vi "ProfilerTest.vi"() -> ()   [LabVIEW 2014] (continued)
{35.59000000000149, 1.3677623388053117e-07}, {35.60000000000149, 1.3677623388053117e-07}, {35.610000000001484, 1.3677623388053117e-07}, {35.62000000000148, 1.3677623388053117e-07}, {35.63000000000148, 1.3677623388053117e-07}, {35.64000000000148, 1.3677623388053117e-07}, {35.65000000000148, 1.3677623388053117e-07}, {35.660000000001475, 1.3677623388053117e-07}, {35.67000000000147, 1.3677623388053117e-07}, {35.68000000000147, 1.3677623388053117e-07}, {35.69000000000147, 1.3677623388053117e-07}, {35.70000000000147, 1.3677623388053117e-07}, {35.710000000001465, 1.3677623388053117e-07}, {35.72000000000146, 1.3677623388053117e-07}, {35.73000000000146, 1.3677623388053117e-07}, {35.74000000000146, 1.3677623388053117e-07}, {35.75000000000146, 1.3677623388053117e-07}, {35.760000000001455, 1.3677623388053117e-07}, {35.77000000000145, 1.3677623388053117e-07}, {35.78000000000145, 1.3677623388053117e-07}, {35.79000000000145, 1.3677623388053117e-07}, {35.80000000000145, 1.3677623388053117e-07}, {35.810000000001445, 1.3677623388053117e-07}, {35.82000000000144, 1.3677623388053117e-07}, {35.83000000000144, 1.3677623388053117e-07}, {35.84000000000144, 1.3677623388053117e-07}, {35.85000000000144, 1.3677623388053117e-07}, {35.860000000001435, 1.3677623388053117e-07}, {35.87000000000143, 1.3677623388053117e-07}, {35.88000000000143, 1.3677623388053117e-07}, {35.89000000000143, 1.3677623388053117e-07}, {35.90000000000143, 1.3677623388053117e-07}, {35.910000000001425, 1.3677623388053117e-07}, {35.92000000000142, 1.3677623388053117e-07}, {35.93000000000142, 1.3677623388053117e-07}, {35.94000000000142, 1.3677623388053117e-07}, {35.95000000000142, 1.3677623388053117e-07}, {35.960000000001415, 1.3677623388053117e-07}, {35.97000000000141, 1.3677623388053117e-07}, {35.98000000000141, 1.3677623388053117e-07}, {35.99000000000141, 1.3677623388053117e-07}, {36.00000000000141, 1.3677623388053117e-07}, {36.010000000001405, 1.3677623388053117e-07}, {36.0200000000014, 1.3677623388053117e-07}, {36.0300000000014, 1.3677623388053117e-07}, {36.0400000000014, 1.3677623388053117e-07}, {36.0500000000014, 1.3677623388053117e-07}, {36.060000000001395, 1.3677623388053117e-07}, {36.07000000000139, 1.3677623388053117e-07}, {36.08000000000139, 1.3677623388053117e-07}, {36.09000000000139, 1.3677623388053117e-07}, {36.10000000000139, 1.3677623388053117e-07}, {36.110000000001385, 1.3677623388053117e-07}, {36.12000000000138, 1.3677623388053117e-07}, {36.13000000000138, 1.3677623388053117e-07}, {36.14000000000138, 1.3677623388053117e-07}, {36.15000000000138, 1.3677623388053117e-07}, {36.160000000001375, 1.3677623388053117e-07}, {36.17000000000137, 1.3677623388053117e-07}, {36.18000000000137, 1.3677623388053117e-07}, {36.19000000000137, 1.3677623388053117e-07}, {36.20000000000137, 1.3677623388053117e-07}, {36.210000000001365, 1.3677623388053117e-07}, {36.22000000000136, 1.3677623388053117e-07}, {36.23000000000136, 1.3677623388053117e-07}, {36.24000000000136, 1.3677623388053117e-07}, {36.25000000000136, 1.3677623388053117e-07}, {36.260000000001355, 1.3677623388053117e-07}, {36.27000000000135, 1.3677623388053117e-07}, {36.28000000000135, 1.3677623388053117e-07}, {36.29000000000135, 1.3677623388053117e-07}, {36.30000000000135, 1.3677623388053117e-07}, {36.310000000001345, 1.3677623388053117e-07}, {36.32000000000134, 1.3677623388053117e-07}, {36.33000000000134, 1.3677623388053117e-07}, {36.34000000000134, 1.3677623388053117e-07}, {36.35000000000134, 1.3677623388053117e-07}, {36.360000000001335, 1.3677623388053117e-07}, {36.37000000000133, 1.3677623388053117e-07}, {36.38000000000133, 1.3677623388053117e-07}, {36.39000000000133, 1.3677623388053117e-07}, {36.40000000000133, 1.3677623388053117e-07}, {36.410000000001325, 1.3677623388053117e-07}, {36.42000000000132, 1.3677623388053117e-07}, {36.43000000000132, 1.3677623388053117e-07}, {36.44000000000132, 1.3677623388053117e-07}, {36.45000000000132, 1.3677623388053117e-07}, {36.460000000001315, 1.3677623388053117e-07}, {36.47000000000131, 1.3677623388053117e-07}, {36.48000000000131, 1.3677623388053117e-07}, {36.49000000000131, 1.3677623388053117e-07}, {36.50000000000131, 1.3677623388053117e-07}, {36.510000000001305, 1.3677623388053117e-07}, {36.5200000000013, 1.3677623388053117e-07}, {36.5300000000013, 1.3677623388053117e-07}, {36.5400000000013, 1.3677623388053117e-07}, {36.5500000000013, 1.3677623388053117e-07}, {36.560000000001295, 1.3677623388053117e-07}, {36.57000000000129, 1.3677623388053117e-07}, {36.58000000000129, 1.3677623388053117e-07}, {36.59000000000129, 1.3677623388053117e-07}, {36.60000000000129, 1.3677623388053117e-07}, {36.610000000001286, 1.3677623388053117e-07}, {36.62000000000128, 1.3677623388053117e-07}, {36.63000000000128, 1.3677623388053117e-07}, {36.64000000000128, 1.3677623388053117e-07}, {36.65000000000128, 1.3677623388053117e-07}, {36.660000000001276, 1.3677623388053117e-07}, {36.670000000001274, 1.3677623388053117e-07}, {36.68000000000127, 1.3677623388053117e-07}, {36.69000000000127, 1.3677623388053117e-07}, {36.70000000000127, 1.3677623388053117e-07}, {36.710000000001266, 1.3677623388053117e-07}, {36.720000000001264, 1.3677623388053117e-07}, {36.73000000000126, 1.3677623388053117e-07}, {36.74000000000126, 1.3677623388053117e-07}, {36.75000000000126, 1.3677623388053117e-07}, {36.760000000001256, 1.3677623388053117e-07}, {36.770000000001254, 1.3677623388053117e-07}, {36.78000000000125, 1.3677623388053117e-07}, {36.79000000000125, 1.3677623388053117e-07}, {36.80000000000125, 1.3677623388053117e-07}, {36.810000000001246, 1.3677623388053117e-07}, {36.820000000001244, 1.3677623388053117e-07}, {36.83000000000124, 1.3677623388053117e-07}, {36.84000000000124, 1.3677623388053117e-07}, {36.85000000000124, 1.3677623388053117e-07}, {36.860000000001236, 1.3677623388053117e-07}, {36.870000000001234, 1.3677623388053117e-07}, {36.88000000000123, 1.3677623388053117e-07}, {36.89000000000123, 1.3677623388053117e-07}, {36.90000000000123, 1.3677623388053117e-07}, {36.910000000001226, 1.3677623388053117e-07}, {36.920000000001224, 1.3677623388053117e-07}, {36.93000000000122, 1.3677623388053117e-07}, {36.94000000000122, 1.3677623388053117e-07}, {36.95000000000122, 1.3677623388053117e-07}, {36.960000000001216, 1.3677623388053117e-07}, {36.970000000001214, 1.3677623388053117e-07}, {36.98000000000121, 1.3677623388053117e-07}, {36.99000000000121, 1.3677623388053117e-07}, {37.00000000000121, 1.3677623388053117e-07}, {37.010000000001206, 1.3677623388053117e-07}, {37.020000000001204, 1.3677623388053117e-07}, {37.0300000000012, 1.3677623388053117e-07}, {37.0400000000012, 1.3677623388053117e-07}, {37.0500000000012, 1.3677623388053117e-07}, {37.060000000001196, 1.3677623388053117e-07}, {37.070000000001194, 1.3677623388053117e-07}, {37.08000000000119, 1.3677623388053117e-07}, {37.09000000000119, 1.3677623388053117e-07}, {37.10000000000119, 1.3677623388053117e-07}, {37.110000000001186, 1.3677623388053117e-07}, {37.120000000001184, 1.3677623388053117e-07}, {37.13000000000118, 1.3677623388053117e-07}, {37.14000000000118, 1.3677623388053117e-07}, {37.15000000000118, 1.3677623388053117e-07}, {37.160000000001176, 1.3677623388053117e-07}, {37.170000000001174, 1.3677623388053117e-07}, {37.18000000000117, 1.3677623388053117e-07}, {37.19000000000117, 1.3677623388053117e-07}, {37.20000000000117, 1.3677623388053117e-07}, {37.210000000001166, 1.3677623388053117e-07}, {37.220000000001164, 1.3677623388053117e-07}, {37.23000000000116, 1.3677623388053117e-07}, {37.24000000000116, 1.3677623388053117e-07}, {37.25000000000116, 1.3677623388053117e-07}, {37.260000000001156, 1.3677623388053117e-07}, {37.270000000001154, 1.3677623388053117e-07}, {37.28000000000115, 1.3677623388053117e-07}, {37.29000000000115, 1.3677623388053117e-07}, {37.30000000000115, 1.3677623388053117e-07}, {37.310000000001146, 1.3677623388053117e-07}, {37.320000000001144, 1.3677623388053117e-07}, {37.33000000000114, 1.3677623388053117e-07}, {37.34000000000114, 1.3677623388053117e-07}, {37.35000000000114, 1.3677623388053117e-07}, {37.360000000001136, 1.3677623388053117e-07}, {37.370000000001134, 1.3677623388053117e-07}, {37.38000000000113, 1.3677623388053117e-07}, {37.39000000000113, 1.3677623388053117e-07}, {37.40000000000113, 1.3677623388053117e-07}, {37.410000000001126, 1.3677623388053117e-07}, {37.420000000001124, 1.3677623388053117e-07}, {37.43000000000112, 1.3677623388053117e-07}, {37.44000000000112, 1.3677623388053117e-07}, {37.45000000000112, 1.3677623388053117e-07}, {37.460000000001116, 1.3677623388053117e-07}, {37.470000000001114, 1.3677623388053117e-07}, {37.48000000000111, 1.3677623388053117e-07}, {37.49000000000111, 1.3677623388053117e-07}, {37.50000000000111, 1.3677623388053117e-07}, {37.51000000000111, 1.3677623388053117e-07}, {37.520000000001104, 1.3677623388053117e-07}, {37.5300000000011, 1.3677623388053117e-07}, {37.5400000000011, 1.3677623388053117e-07}, {37.5500000000011, 1.3677623388053117e-07}, {37.5600000000011, 1.3677623388053117e-07}, {37.570000000001095, 1.3677623388053117e-07}, {37.58000000000109, 1.3677623388053117e-07}, {37.59000000000109, 1.3677623388053117e-07}, {37.60000000000109, 1.3677623388053117e-07}, {37.61000000000109, 1.3677623388053117e-07}, {37.620000000001085, 1.3677623388053117e-07}, {37.63000000000108, 1.3677623388053117e-07}, {37.64000000000108, 1.3677623388053117e-07}, {37.65000000000108, 1.3677623388053117e-07}, {37.66000000000108, 1.3677623388053117e-07}, {37.670000000001075, 1.3677623388053117e-07}, {37.68000000000107, 1.3677623388053117e-07}, {37.69000000000107, 1.3677623388053117e-07}, {37.70000000000107, 1.3677623388053117e-07}, {37.71000000000107, 1.3677623388053117e-07}, {37.720000000001065, 1.3677623388053117e-07}, {37.73000000000106, 1.3677623388053117e-07}, {37.74000000000106, 1.3677623388053117e-07}, {37.75000000000106, 1.3677623388053117e-07}, {37.76000000000106, 1.3677623388053117e-07}, {37.770000000001055, 1.3677623388053117e-07}, {37.78000000000105, 1.3677623388053117e-07}, {37.79000000000105, 1.3677623388053117e-07}, {37.80000000000105, 1.3677623388053117e-07}, {37.81000000000105, 1.3677623388053117e-07}, {37.820000000001045, 1.3677623388053117e-07}, {37.83000000000104, 1.3677623388053117e-07}, {37.84000000000104, 1.3677623388053117e-07}, {37.85000000000104, 1.3677623388053117e-07}, {37.86000000000104, 1.3677623388053117e-07}, {37.870000000001035, 1.3677623388053117e-07}, {37.88000000000103, 1.3677623388053117e-07}, {37.89000000000103, 1.3677623388053117e-07}, {37.90000000000103, 1.3677623388053117e-07}, {37.91000000000103, 1.3677623388053117e-07}, {37.920000000001025, 1.3677623388053117e-07}, {37.93000000000102, 1.3677623388053117e-07}, {37.94000000000102, 1.3677623388053117e-07}, {37.95000000000102, 1.3677623388053117e-07}, {37.96000000000102, 1.3677623388053117e-07}, {37.970000000001015, 1.3677623388053117e-07}, {37.98000000000101, 1.3677623388053117e-07}, {37.99000000000101, 1.3677623388053117e-07}, {38.00000000000101, 1.3677623388053117e-07}, {38.01000000000101, 1.3677623388053117e-07}, {38.020000000001005, 1.3677623388053117e-07}, {38.030000000001, 1.3677623388053117e-07}, {38.040000000001, 1.3677623388053117e-07}, {38.050000000001, 1.3677623388053117e-07}, {38.060000000001, 1.3677623388053117e-07}, {38.070000000000995, 1.3677623388053117e-07}, {38.08000000000099, 1.3677623388053117e-07}, {38.09000000000099, 1.3677623388053117e-07}, {38.10000000000099, 1.3677623388053117e-07}, {38.11000000000099, 1.3677623388053117e-07}, {38.120000000000985, 1.3677623388053117e-07}, {38.13000000000098, 1.3677623388053117e-07}, {38.14000000000098, 1.3677623388053117e-07}, {38.15000000000098, 1.3677623388053117e-07}, {38.16000000000098, 1.3677623388053117e-07}, {38.170000000000975, 1.3677623388053117e-07}, {38.18000000000097, 1.3677623388053117e-07}, {38.19000000000097, 1.3677623388053117e-07}, {38.20000000000097, 1.3677623388053117e-07}, {38.21000000000097, 1.3677623388053117e-07}, {38.220000000000965, 1.3677623388053117e-07}, {38.23000000000096, 1.3677623388053117e-07}, {38.24000000000096, 1.3677623388053117e-07}, {38.25000000000096, 1.3677623388053117e-07}, {38.26000000000096, 1.3677623388053117e-07}, {38.270000000000955, 1.3677623388053117e-07}, {38.28000000000095, 1.3677623388053117e-07}, {38.29000000000095, 1.3677623388053117e-07}, {38.30000000000095, 1.3677623388053117e-07}, {38.31000000000095, 1.3677623388053117e-07}, {38.320000000000945, 1.3677623388053117e-07}, {38.33000000000094, 1.3677623388053117e-07}, {38.34000000000094, 1.3677623388053117e-07}, {38.35000000000094, 1.3677623388053117e-07}, {38.36000000000094, 1.3677623388053117e-07}, {38.370000000000935, 1.3677623388053117e-07}, {38.38000000000093, 1.3677623388053117e-07}, {38.39000000000093, 1.3677623388053117e-07}, {38.40000000000093, 1.3677623388053117e-07}, {38.41000000000093, 1.3677623388053117e-07}, {38.420000000000925, 1.3677623388053117e-07}, {38.43000000000092, 1.3677623388053117e-07}, {38.44000000000092, 1.3677623388053117e-07}, {38.45000000000092, 1.3677623388053117e-07}, {38.46000000000092, 1.3677623388053117e-07}, {38.470000000000915, 1.3677623388053117e-07}, {38.48000000000091, 1.3677623388053117e-07}, {38.49000000000091, 1.3677623388053117e-07}, {38.50000000000091, 1.3677623388053117e-07}, {38.51000000000091, 1.3677623388053117e-07}, {38.520000000000906, 1.3677623388053117e-07}, {38.5300000000009, 1.3677623388053117e-07}, {38.5400000000009, 1.3677623388053117e-07}, {38.5500000000009, 1.3677623388053117e-07}, {38.5600000000009, 1.3677623388053117e-07}, {38.570000000000896, 1.3677623388053117e-07}, {38.580000000000894, 1.3677623388053117e-07}, {38.59000000000089, 1.3677623388053117e-07}, {38.60000000000089, 1.3677623388053117e-07}, {38.61000000000089, 1.3677623388053117e-07}, {38.620000000000886, 1.3677623388053117e-07}, {38.630000000000884, 1.3677623388053117e-07}, {38.64000000000088, 1.3677623388053117e-07}, {38.65000000000088, 1.3677623388053117e-07}, {38.66000000000088, 1.3677623388053117e-07}, {38.670000000000876, 1.3677623388053117e-07}, {38.680000000000874, 1.3677623388053117e-07}, {38.69000000000087, 1.3677623388053117e-07}, {38.70000000000087, 1.3677623388053117e-07}, {38.71000000000087, 1.3677623388053117e-07}, {38.720000000000866, 1.3677623388053117e-07}, {38.730000000000864, 1.3677623388053117e-07}, {38.74000000000086, 1.3677623388053117e-07}, {38.75000000000086, 1.3677623388053117e-07}, {38.76000000000086, 1.3677623388053117e-07}, {38.770000000000856, 1.3677623388053117e-07}, {38.780000000000854, 1.3677623388053117e-07}, {38.79000000000085, 1.3677623388053117e-07}, {38.80000000000085, 1.3677623388053117e-07}, {38.81000000000085, 1.3677623388053117e-07}, {38.820000000000846, 1.3677623388053117e-07}, {38.830000000000844, 1.3677623388053117e-07}, {38.84000000000084, 1.3677623388053117e-07}, {38.85000000000084, 1.3677623388053117e-07}, {38.86000000000084, 1.3677623388053117e-07}, {38.870000000000836, 1.3677623388053117e-07}, {38.880000000000834, 1.3677623388053117e-07}, {38.89000000000083, 1.3677623388053117e-07}, {38.90000000000083, 1.3677623388053117e-07}, {38.91000000000083, 1.3677623388053117e-07}, {38.920000000000826, 1.3677623388053117e-07}, {38.930000000000824, 1.3677623388053117e-07}, {38.94000000000082, 1.3677623388053117e-07}, {38.95000000000082, 1.3677623388053117e-07}, {38.96000000000082, 1.3677623388053117e-07}, {38.970000000000816, 1.3677623388053117e-07}, {38.980000000000814, 1.3677623388053117e-07}, {38.99000000000081, 1.3677623388053117e-07}, {39.00000000000081, 1.3677623388053117e-07}, {39.01000000000081, 1.3677623388053117e-07}, {39.020000000000806, 1.3677623388053117e-07}, {39.030000000000804, 1.3677623388053117e-07}, {39.0400000000008, 1.3677623388053117e-07}, {39.0500000000008, 1.3677623388053117e-07}, {39.0600000000008, 1.3677623388053117e-07}, {39.070000000000796, 1.3677623388053117e-07}, {39.080000000000794, 1.3677623388053117e-07}, {39.09000000000079, 1.3677623388053117e-07}, {39.10000000000079, 1.3677623388053117e-07}, {39.11000000000079, 1.3677623388053117e-07}, {39.120000000000786, 1.3677623388053117e-07}, {39.130000000000784, 1.3677623388053117e-07}, {39.14000000000078, 1.3677623388053117e-07}, {39.15000000000078, 1.3677623388053117e-07}, {39.16000000000078, 1.3677623388053117e-07}, {39.170000000000776, 1.3677623388053117e-07}, {39.180000000000774, 1.3677623388053117e-07}, {39.19000000000077, 1.3677623388053117e-07}, {39.20000000000077, 1.3677623388053117e-07}, {39.21000000000077, 1.3677623388053117e-07}, {39.220000000000766, 1.3677623388053117e-07}, {39.230000000000764, 1.3677623388053117e-07}, {39.24000000000076, 1.3677623388053117e-07}, {39.25000000000076, 1.3677623388053117e-07}, {39.26000000000076, 1.3677623388053117e-07}, {39.270000000000756, 1.3677623388053117e-07}, {39.280000000000754, 1.3677623388053117e-07}, {39.29000000000075, 1.3677623388053117e-07}, {39.30000000000075, 1.3677623388053117e-07}, {39.31000000000075, 1.3677623388053117e-07}, {39.320000000000746, 1.3677623388053117e-07}, {39.330000000000744, 1.3677623388053117e-07}, {39.34000000000074, 1.3677623388053117e-07}, {39.35000000000074, 1.3677623388053117e-07}, {39.36000000000074, 1.3677623388053117e-07}, {39.370000000000736, 1.3677623388053117e-07}, {39.380000000000734, 1.3677623388053117e-07}, {39.39000000000073, 1.3677623388053117e-07}, {39.40000000000073, 1.3677623388053117e-07}, {39.41000000000073, 1.3677623388053117e-07}, {39.42000000000073, 1.3677623388053117e-07}, {39.430000000000724, 1.3677623388053117e-07}, {39.44000000000072, 1.3677623388053117e-07}, {39.45000000000072, 1.3677623388053117e-07}, {39.46000000000072, 1.3677623388053117e-07}, {39.47000000000072, 1.3677623388053117e-07}, {39.480000000000715, 1.3677623388053117e-07}, {39.49000000000071, 1.3677623388053117e-07}, {39.50000000000071, 1.3677623388053117e-07}, {39.51000000000071, 1.3677623388053117e-07}, {39.52000000000071, 1.3677623388053117e-07}, {39.530000000000705, 1.3677623388053117e-07}, {39.5400000000007, 1.3677623388053117e-07}, {39.5500000000007, 1.3677623388053117e-07}, {39.5600000000007, 1.3677623388053117e-07}, {39.5700000000007, 1.3677623388053117e-07}, {39.580000000000695, 1.3677623388053117e-07}, {39.59000000000069, 1.3677623388053117e-07}, {39.60000000000069, 1.3677623388053117e-07}, {39.61000000000069, 1.3677623388053117e-07}, {39.62000000000069, 1.3677623388053117e-07}, {39.630000000000685, 1.3677623388053117e-07}, {39.64000000000068, 1.3677623388053117e-07}, {39.65000000000068, 1.3677623388053117e-07}, {39.66000000000068, 1.3677623388053117e-07}, {39.67000000000068, 1.3677623388053117e-07}, {39.680000000000675, 1.3677623388053117e-07}, {39.69000000000067, 1.3677623388053117e-07}, {39.70000000000067, 1.3677623388053117e-07}, {39.71000000000067, 1.3677623388053117e-07}, {39.72000000000067, 1.3677623388053117e-07}, {39.730000000000665, 1.3677623388053117e-07}, {39.74000000000066, 1.3677623388053117e-07}, {39.75000000000066, 1.3677623388053117e-07}, {39.76000000000066, 1.3677623388053117e-07}, {39.77000000000066, 1.3677623388053117e-07}, {39.780000000000655, 1.3677623388053117e-07}, {39.79000000000065, 1.3677623388053117e-07}, {39.80000000000065, 1.3677623388053117e-07}, {39.81000000000065, 1.3677623388053117e-07}, {39.82000000000065, 1.3677623388053117e-07}, {39.830000000000645, 1.3677623388053117e-07}, {39.84000000000064, 1.3677623388053117e-07}, {39.85000000000064, 1.3677623388053117e-07}, {39.86000000000064, 1.3677623388053117e-07}, {39.87000000000064, 1.3677623388053117e-07}, {39.880000000000635, 1.3677623388053117e-07}, {39.89000000000063, 1.3677623388053117e-07}, {39.90000000000063, 1.3677623388053117e-07}, {39.91000000000063, 1.3677623388053117e-07}, {39.92000000000063, 1.3677623388053117e-07}, {39.930000000000625, 1.3677623388053117e-07}, {39.94000000000062, 1.3677623388053117e-07}, {39.95000000000062, 1.3677623388053117e-07}, {39.96000000000062, 1.3677623388053117e-07}, {39.97000000000062, 1.3677623388053117e-07}, {39.980000000000615, 1.3677623388053117e-07}, {39.99000000000061, 1.3677623388053117e-07}, {0.0, 0.0}]}, ...(2 in all)]
  out "VelocityProfile":T3(graph)=[{[{"Time"=0.0, "delVelocity"=0.0}, {"Time"=0.5, "delVelocity"=0.0}, {"Time"=0.5, "delVelocity"=0.7071067811865475}, {"Time"=1.2071067811865475, "delVelocity"=0.7071067811865475}, {"Time"=1.2071067811865475, "delVelocity"=0.7071067811865475}, {"Time"=1.914213562373095, "delVelocity"=0.7071067811865475}, {"Time"=1.914213562373095, "delVelocity"=-0.7071067811865475}, {"Time"=2.6213203435596424, "delVelocity"=-0.7071067811865475}, {"Time"=2.6213203435596424, "delVelocity"=-0.7071067811865475}, {"Time"=3.32842712474619, "delVelocity"=-0.7071067811865475}, {"Time"=3.32842712474619, "delVelocity"=0.0}, {"Time"=3.82842712474619, "delVelocity"=0.0}]}, {[{"Time"=0.0, "delVelocity"=1.0}, {"Time"=0.5, "delVelocity"=1.0}, {"Time"=0.5, "delVelocity"=0.7071067811865475}, {"Time"=1.2071067811865475, "delVelocity"=0.7071067811865475}, {"Time"=1.2071067811865475, "delVelocity"=-0.7071067811865475}, {"Time"=1.914213562373095, "delVelocity"=-0.7071067811865475}, {"Time"=1.914213562373095, "delVelocity"=-0.7071067811865475}, {"Time"=2.6213203435596424, "delVelocity"=-0.7071067811865475}, {"Time"=2.6213203435596424, "delVelocity"=0.7071067811865475}, {"Time"=3.32842712474619, "delVelocity"=0.7071067811865475}, {"Time"=3.32842712474619, "delVelocity"=-1.0}, {"Time"=3.82842712474619, "delVelocity"=-1.0}]}, {[{"Time"=0.01, "delVelocity"=0.0}, {"Time"=0.02, "delVelocity"=0.0}, {"Time"=0.03, "delVelocity"=0.0}, {"Time"=0.04, "delVelocity"=0.0}, {"Time"=0.05, "delVelocity"=0.0}, {"Time"=0.060000000000000005, "delVelocity"=0.0}, {"Time"=0.07, "delVelocity"=0.0}, {"Time"=0.08, "delVelocity"=0.0}, {"Time"=0.09, "delVelocity"=0.0}, {"Time"=0.09999999999999999, "delVelocity"=0.0}, {"Time"=0.10999999999999999, "delVelocity"=0.0}, {"Time"=0.11999999999999998, "delVelocity"=0.0}, {"Time"=0.12999999999999998, "delVelocity"=0.0}, {"Time"=0.13999999999999999, "delVelocity"=0.0}, {"Time"=0.15, "delVelocity"=0.0}, {"Time"=0.16, "delVelocity"=0.0}, {"Time"=0.17, "delVelocity"=0.0}, {"Time"=0.18000000000000002, "delVelocity"=0.0}, {"Time"=0.19000000000000003, "delVelocity"=0.0}, {"Time"=0.20000000000000004, "delVelocity"=0.0}, {"Time"=0.21000000000000005, "delVelocity"=0.0}, {"Time"=0.22000000000000006, "delVelocity"=0.0}, {"Time"=0.23000000000000007, "delVelocity"=0.0}, {"Time"=0.24000000000000007, "delVelocity"=0.0}, {"Time"=0.25000000000000006, "delVelocity"=0.0}, {"Time"=0.26000000000000006, "delVelocity"=0.0}, {"Time"=0.2700000000000001, "delVelocity"=0.0}, {"Time"=0.2800000000000001, "delVelocity"=0.0}, {"Time"=0.2900000000000001, "delVelocity"=0.0}, {"Time"=0.3000000000000001, "delVelocity"=0.0}, {"Time"=0.3100000000000001, "delVelocity"=0.0}, {"Time"=0.3200000000000001, "delVelocity"=0.0}, {"Time"=0.3300000000000001, "delVelocity"=0.0}, {"Time"=0.34000000000000014, "delVelocity"=0.0}, {"Time"=0.35000000000000014, "delVelocity"=0.0}, {"Time"=0.36000000000000015, "delVelocity"=3.652435472123461e-09}, {"Time"=0.37000000000000016, "delVelocity"=2.935262808090311e-05}, {"Time"=0.38000000000000017, "delVelocity"=0.0005452673769502404}, {"Time"=0.3900000000000002, "delVelocity"=0.0025117876941350113}, {"Time"=0.4000000000000002, "delVelocity"=0.006891877535090485}, {"Time"=0.4100000000000002, "delVelocity"=0.014541665215472843}, {"Time"=0.4200000000000002, "delVelocity"=0.02617254725134448}, {"Time"=0.4300000000000002, "delVelocity"=0.042319698691609564}, {"Time"=0.4400000000000002, "delVelocity"=0.06331838381957455}, {"Time"=0.45000000000000023, "delVelocity"=0.08928911582046334}, {"Time"=0.46000000000000024, "delVelocity"=0.12013232231596303}, {"Time"=0.47000000000000025, "delVelocity"=0.1555327528936659}, {"Time"=0.48000000000000026, "delVelocity"=0.19497343353398233}, {"Time"=0.49000000000000027, "delVelocity"=0.237758550247669}, {"Time"=0.5000000000000002, "delVelocity"=0.28304424898939734}, {"Time"=0.5100000000000002, "delVelocity"=0.32987598850213584}, {"Time"=0.5200000000000002, "delVelocity"=0.3772307926844132}, {"Time"=0.5300000000000002, "delVelocity"=0.4240625321971534}, {"Time"=0.5400000000000003, "delVelocity"=0.4693482309388819}, {"Time"=0.5500000000000003, "delVelocity"=0.5121333476525676}, {"Time"=0.5600000000000003, "delVelocity"=0.5515740282928845}, {"Time"=0.5700000000000003, "delVelocity"=0.5869744588705872}, {"Time"=0.5800000000000003, "delVelocity"=0.6178176653660855}, {"Time"=0.5900000000000003, "delVelocity"=0.6437883973669768}, {"Time"=0.6000000000000003, "delVelocity"=0.6647870824949387}, {"Time"=0.6100000000000003, "delVelocity"=0.6809342339352042}, {"Time"=0.6200000000000003, "delVelocity"=0.6925651159710763}, {"Time"=0.6300000000000003, "delVelocity"=0.7002149036514582}, {"Time"=0.6400000000000003, "delVelocity"=0.7045949934924134}, {"Time"=0.6500000000000004, "delVelocity"=0.7065615138095976}, {"Time"=0.6600000000000004, "delVelocity"=0.7070774249060385}, {"Time"=0.6700000000000004, "delVelocity"=0.7071067811865506}, {"Time"=0.6800000000000004, "delVelocity"=0.7071067811865506}, {"Time"=0.6900000000000004, "delVelocity"=0.7071067811865506}, {"Time"=0.7000000000000004, "delVelocity"=0.7071067811865395}, {"Time"=0.7100000000000004, "delVelocity"=0.7071067811865506}, {"Time"=0.7200000000000004, "delVelocity"=0.7071067811865506}, {"Time"=0.7300000000000004, "delVelocity"=0.7071067811865506}, {"Time"=0.7400000000000004, "delVelocity"=0.7071067811865395}, {"Time"=0.7500000000000004, "delVelocity"=0.7071067811865506}, {"Time"=0.7600000000000005, "delVelocity"=0.7071067811865506}, {"Time"=0.7700000000000005, "delVelocity"=0.7071067811865506}, {"Time"=0.7800000000000005, "delVelocity"=0.7071067811865395}, {"Time"=0.7900000000000005, "delVelocity"=0.7071067811865506}, {"Time"=0.8000000000000005, "delVelocity"=0.7071067811865506}, {"Time"=0.8100000000000005, "delVelocity"=0.7071067811865506}, {"Time"=0.8200000000000005, "delVelocity"=0.7071067811865506}, {"Time"=0.8300000000000005, "delVelocity"=0.7071067811865395}, {"Time"=0.8400000000000005, "delVelocity"=0.7071067811865506}, {"Time"=0.8500000000000005, "delVelocity"=0.7071067811865506}, {"Time"=0.8600000000000005, "delVelocity"=0.7071067811865506}, {"Time"=0.8700000000000006, "delVelocity"=0.7071067811865395}, {"Time"=0.8800000000000006, "delVelocity"=0.7071067811865506}, {"Time"=0.8900000000000006, "delVelocity"=0.7071067811865506}, {"Time"=0.9000000000000006, "delVelocity"=0.7071067811865506}, {"Time"=0.9100000000000006, "delVelocity"=0.7071067811865506}, {"Time"=0.9200000000000006, "delVelocity"=0.7071067811865395}, {"Time"=0.9300000000000006, "delVelocity"=0.7071067811865506}, {"Time"=0.9400000000000006, "delVelocity"=0.7071067811865506}, {"Time"=0.9500000000000006, "delVelocity"=0.707106781186545}, {"Time"=0.9600000000000006, "delVelocity"=0.7071067811865506}, {"Time"=0.9700000000000006, "delVelocity"=0.707106781186545}, {"Time"=0.9800000000000006, "delVelocity"=0.7071067811865506}, {"Time"=0.9900000000000007, "delVelocity"=0.7071067811865506}, {"Time"=1.0000000000000007, "delVelocity"=0.707106781186545}, {"Time"=1.0100000000000007, "delVelocity"=0.7071067811865506}, {"Time"=1.0200000000000007, "delVelocity"=0.707106781186545}, {"Time"=1.0300000000000007, "delVelocity"=0.7071067811865506}, {"Time"=1.0400000000000007, "delVelocity"=0.707106781186545}, {"Time"=1.0500000000000007, "delVelocity"=0.7071067811865506}, {"Time"=1.0600000000000007, "delVelocity"=0.707106781186545}, {"Time"=1.0700000000000007, "delVelocity"=0.7071067811865506}, {"Time"=1.0800000000000007, "delVelocity"=0.7071067811865506}, {"Time"=1.0900000000000007, "delVelocity"=0.707106781186545}, {"Time"=1.1000000000000008, "delVelocity"=0.7071067811865506}, {"Time"=1.1100000000000008, "delVelocity"=0.707106781186545}, {"Time"=1.1200000000000008, "delVelocity"=0.7071067811865506}, {"Time"=1.1300000000000008, "delVelocity"=0.707106781186545}, {"Time"=1.1400000000000008, "delVelocity"=0.7071067811865506}, {"Time"=1.1500000000000008, "delVelocity"=0.707106781186545}, {"Time"=1.1600000000000008, "delVelocity"=0.7071067811865506}, {"Time"=1.1700000000000008, "delVelocity"=0.7071067811865506}, {"Time"=1.1800000000000008, "delVelocity"=0.707106781186545}, {"Time"=1.1900000000000008, "delVelocity"=0.7071067811865506}, {"Time"=1.2000000000000008, "delVelocity"=0.707106781186545}, {"Time"=1.2100000000000009, "delVelocity"=0.7071067811865506}, {"Time"=1.2200000000000009, "delVelocity"=0.7071067811865395}, {"Time"=1.2300000000000009, "delVelocity"=0.7071067811865506}, {"Time"=1.2400000000000009, "delVelocity"=0.7071067811865506}, {"Time"=1.2500000000000009, "delVelocity"=0.7071067811865506}, {"Time"=1.260000000000001, "delVelocity"=0.7071067811865506}, {"Time"=1.270000000000001, "delVelocity"=0.7071067811865506}, {"Time"=1.280000000000001, "delVelocity"=0.7071067811865506}, {"Time"=1.290000000000001, "delVelocity"=0.7071067811865395}, {"Time"=1.300000000000001, "delVelocity"=0.7071067811865506}, {"Time"=1.310000000000001, "delVelocity"=0.7071067811865506}, {"Time"=1.320000000000001, "delVelocity"=0.7071067811865395}, {"Time"=1.330000000000001, "delVelocity"=0.7071067811865506}, {"Time"=1.340000000000001, "delVelocity"=0.7071067811865506}, {"Time"=1.350000000000001, "delVelocity"=0.7071067811865506}, {"Time"=1.360000000000001, "delVelocity"=0.7071067811865506}, {"Time"=1.370000000000001, "delVelocity"=0.7071067811865395}, {"Time"=1.380000000000001, "delVelocity"=0.7071067811865506}, {"Time"=1.390000000000001, "delVelocity"=0.7071067811865506}, {"Time"=1.400000000000001, "delVelocity"=0.7071067811865506}, {"Time"=1.410000000000001, "delVelocity"=0.7071067811865395}, {"Time"=1.420000000000001, "delVelocity"=0.7071067811865506}, {"Time"=1.430000000000001, "delVelocity"=0.7071067811865506}, {"Time"=1.440000000000001, "delVelocity"=0.7071067811865506}, {"Time"=1.450000000000001, "delVelocity"=0.7071067811865506}, {"Time"=1.460000000000001, "delVelocity"=0.7071067811865395}, {"Time"=1.470000000000001, "delVelocity"=0.7071067811865506}, {"Time"=1.480000000000001, "delVelocity"=0.7071067811865506}, {"Time"=1.490000000000001, "delVelocity"=0.7071067811865506}, {"Time"=1.500000000000001, "delVelocity"=0.7071067811865395}, {"Time"=1.5100000000000011, "delVelocity"=0.7071067811865506}, {"Time"=1.5200000000000011, "delVelocity"=0.7071067811865506}, {"Time"=1.5300000000000011, "delVelocity"=0.7071067811865506}, {"Time"=1.5400000000000011, "delVelocity"=0.7071067811865506}, {"Time"=1.5500000000000012, "delVelocity"=0.7071067811865395}, {"Time"=1.5600000000000012, "delVelocity"=0.7071067811865506}, {"Time"=1.5700000000000012, "delVelocity"=0.7071067811865506}, {"Time"=1.5800000000000012, "delVelocity"=0.7071067811865506}, {"Time"=1.5900000000000012, "delVelocity"=0.7071067811865395}, {"Time"=1.6000000000000012, "delVelocity"=0.7071067811865506}, {"Time"=1.6100000000000012, "delVelocity"=0.7071067811865506}, {"Time"=1.6200000000000012, "delVelocity"=0.7071067811865506}, {"Time"=1.6300000000000012, "delVelocity"=0.7071067811865506}, {"Time"=1.6400000000000012, "delVelocity"=0.7071067766482253}, {"Time"=1.6500000000000012, "delVelocity"=0.7070996624839343}, {"Time"=1.6600000000000013, "delVelocity"=0.7069593466320523}, {"Time"=1.6700000000000013, "delVelocity"=0.7064009225472123}, {"Time"=1.6800000000000013, "delVelocity"=0.7051231642495548}, {"Time"=1.6900000000000013, "delVelocity"=0.7028337110694505}, {"Time"=1.7000000000000013, "delVelocity"=0.6992526707960911}, {"Time"=1.7100000000000013, "delVelocity"=0.6941160691606219}, {"Time"=1.7200000000000013, "delVelocity"=0.6871791031415109}, {"Time"=1.7300000000000013, "delVelocity"=0.6782191579970176}, {"Time"=1.7400000000000013, "delVelocity"=0.6670385508421472}, {"Time"=1.7500000000000013, "delVelocity"=0.6534669669571835}, {"Time"=1.7600000000000013, "delVelocity"=0.6373635588020954}, {"Time"=1.7700000000000014, "delVelocity"=0.6186186818676775}, {"Time"=1.7800000000000014, "delVelocity"=0.5971552459703044}, {"Time"=1.7900000000000014, "delVelocity"=0.5729296653367189}, {"Time"=1.8000000000000014, "delVelocity"=0.5459323957691553}, {"Time"=1.8100000000000014, "delVelocity"=0.5161880522714268}, {"Time"=1.8200000000000014, "delVelocity"=0.4837551056852907}, {"Time"=1.8300000000000014, "delVelocity"=0.4487251620768462}, {"Time"=1.8400000000000014, "delVelocity"=0.4112218337533613}, {"Time"=1.8500000000000014, "delVelocity"=0.3713992158246415}, {"Time"=1.8600000000000014, "delVelocity"=0.3294399870846565}, {"Time"=1.8700000000000014, "delVelocity"=0.2855531586180904}, {"Time"=1.8800000000000014, "delVelocity"=0.2399714978795653}, {"Time"=1.8900000000000015, "delVelocity"=0.1929486599911323}, {"Time"=1.9000000000000015, "delVelocity"=0.14475606161371557}, {"Time"=1.9100000000000015, "delVelocity"=0.09567953591929079}, {"Time"=1.9200000000000015, "delVelocity"=0.04601580988929932}, {"Time"=1.9300000000000015, "delVelocity"=-0.003931152645642033}, {"Time"=1.9400000000000015, "delVelocity"=-0.05385389715563127}, {"Time"=1.9500000000000015, "delVelocity"=-0.10344526758157002}, {"Time"=1.9600000000000015, "delVelocity"=-0.15240219182703907}, {"Time"=1.9700000000000015, "delVelocity"=-0.20042941691795768}, {"Time"=1.9800000000000015, "delVelocity"=-0.24724314779684953}, {"Time"=1.9900000000000015, "delVelocity"=-0.2925745449060546}, {"Time"=2.0000000000000013, "delVelocity"=-0.3361730374543015}, {"Time"=2.010000000000001, "delVelocity"=-0.37780941153323644}, {"Time"=2.020000000000001, "delVelocity"=-0.4172786350246649}, {"Time"=2.0300000000000007, "delVelocity"=-0.45440238448331005}, {"Time"=2.0400000000000005, "delVelocity"=-0.4890312428534771}, {"Time"=2.0500000000000003, "delVelocity"=-0.5210465409336673}, {"Time"=2.06, "delVelocity"=-0.5503618198946403}, {"Time"=2.07, "delVelocity"=-0.5769238968263313}, {"Time"=2.0799999999999996, "delVelocity"=-0.600713520181495}, {"Time"=2.0899999999999994, "delVelocity"=-0.621745607037949}, {"Time"=2.099999999999999, "delVelocity"=-0.6400690592557434}, {"Time"=2.109999999999999, "delVelocity"=-0.6557661607946241}, {"Time"=2.1199999999999988, "delVelocity"=-0.6689515636194576}, {"Time"=2.1299999999999986, "delVelocity"=-0.6797708746920872}, {"Time"=2.1399999999999983, "delVelocity"=-0.6883988614633241}, {"Time"=2.149999999999998, "delVelocity"=-0.6950372979818153}, {"Time"=2.159999999999998, "delVelocity"=-0.6999124781645438}, {"Time"=2.1699999999999977, "delVelocity"=-0.7032724268765889}, {"Time"=2.1799999999999975, "delVelocity"=-0.7053838431915316}, {"Time"=2.1899999999999973, "delVelocity"=-0.7065288135048142}, {"Time"=2.199999999999997, "delVelocity"=-0.7070013350085835}, {"Time"=2.209999999999997, "delVelocity"=-0.7071035958776672}, {"Time"=2.2199999999999966, "delVelocity"=-0.7071067811865395}, {"Time"=2.2299999999999964, "delVelocity"=-0.7071067811865284}, {"Time"=2.239999999999996, "delVelocity"=-0.7071067811865284}, {"Time"=2.249999999999996, "delVelocity"=-0.7071067811865395}, {"Time"=2.259999999999996, "delVelocity"=-0.7071067811865284}, {"Time"=2.2699999999999956, "delVelocity"=-0.7071067811865284}, {"Time"=2.2799999999999954, "delVelocity"=-0.7071067811865395}, {"Time"=2.289999999999995, "delVelocity"=-0.7071067811865284}, {"Time"=2.299999999999995, "delVelocity"=-0.7071067811865395}, {"Time"=2.3099999999999947, "delVelocity"=-0.7071067811865284}, {"Time"=2.3199999999999945, "delVelocity"=-0.7071067811865284}, {"Time"=2.3299999999999943, "delVelocity"=-0.7071067811865395}, {"Time"=2.339999999999994, "delVelocity"=-0.7071067811865284}, {"Time"=2.349999999999994, "delVelocity"=-0.7071067811865284}, {"Time"=2.3599999999999937, "delVelocity"=-0.7071067811865395}, {"Time"=2.3699999999999934, "delVelocity"=-0.7071067811865284}, {"Time"=2.3799999999999932, "delVelocity"=-0.7071067811865284}, {"Time"=2.389999999999993, "delVelocity"=-0.7071067811865395}, {"Time"=2.399999999999993, "delVelocity"=-0.7071067811865284}, {"Time"=2.4099999999999926, "delVelocity"=-0.7071067811865284}, {"Time"=2.4199999999999924, "delVelocity"=-0.7071067811865395}, {"Time"=2.429999999999992, "delVelocity"=-0.7071067811865284}, {"Time"=2.439999999999992, "delVelocity"=-0.7071067811865395}, {"Time"=2.4499999999999917, "delVelocity"=-0.7071067811865284}, {"Time"=2.4599999999999915, "delVelocity"=-0.7071067811865284}, {"Time"=2.4699999999999913, "delVelocity"=-0.7071067811865395}, {"Time"=2.479999999999991, "delVelocity"=-0.7071067811865284}, {"Time"=2.489999999999991, "delVelocity"=-0.7071067811865284}, {"Time"=2.4999999999999907, "delVelocity"=-0.7071067811865395}, {"Time"=2.5099999999999905, "delVelocity"=-0.7071067811865284}, {"Time"=2.5199999999999902, "delVelocity"=-0.7071067811865284}, {"Time"=2.52999999999999, "delVelocity"=-0.7071067811865395}, {"Time"=2.53999999999999, "delVelocity"=-0.7071067811865284}, {"Time"=2.5499999999999896, "delVelocity"=-0.7071067811865284}, {"Time"=2.5599999999999894, "delVelocity"=-0.7071067811865395}, {"Time"=2.569999999999989, "delVelocity"=-0.7071067811865284}, {"Time"=2.579999999999989, "delVelocity"=-0.7071067811865284}, {"Time"=2.5899999999999888, "delVelocity"=-0.7071067811865395}, {"Time"=2.5999999999999885, "delVelocity"=-0.7071067811865284}, {"Time"=2.6099999999999883, "delVelocity"=-0.7071067811865284}, {"Time"=2.619999999999988, "delVelocity"=-0.7071067811865395}, {"Time"=2.629999999999988, "delVelocity"=-0.7071067811865284}, {"Time"=2.6399999999999877, "delVelocity"=-0.7071067811865339}, {"Time"=2.6499999999999875, "delVelocity"=-0.7071067811865284}, {"Time"=2.6599999999999873, "delVelocity"=-0.7071067811865339}, {"Time"=2.669999999999987, "delVelocity"=-0.7071067811865339}, {"Time"=2.679999999999987, "delVelocity"=-0.7071067811865339}, {"Time"=2.6899999999999866, "delVelocity"=-0.7071067811865284}, {"Time"=2.6999999999999864, "delVelocity"=-0.7071067811865339}, {"Time"=2.709999999999986, "delVelocity"=-0.7071067811865339}, {"Time"=2.719999999999986, "delVelocity"=-0.7071067811865284}, {"Time"=2.7299999999999858, "delVelocity"=-0.7071067811865339}, {"Time"=2.7399999999999856, "delVelocity"=-0.7071067811865339}, {"Time"=2.7499999999999853, "delVelocity"=-0.7071067811865339}, {"Time"=2.759999999999985, "delVelocity"=-0.7071067811865284}, {"Time"=2.769999999999985, "delVelocity"=-0.7071067811865339}, {"Time"=2.7799999999999847, "delVelocity"=-0.7071067811865339}, {"Time"=2.7899999999999845, "delVelocity"=-0.7071067811865339}, {"Time"=2.7999999999999843, "delVelocity"=-0.7071067811865284}, {"Time"=2.809999999999984, "delVelocity"=-0.7071067811865339}, {"Time"=2.819999999999984, "delVelocity"=-0.7071067811865339}, {"Time"=2.8299999999999836, "delVelocity"=-0.7071067811865284}, {"Time"=2.8399999999999834, "delVelocity"=-0.7071067811865339}, {"Time"=2.849999999999983, "delVelocity"=-0.7071067811865339}, {"Time"=2.859999999999983, "delVelocity"=-0.7071067811865339}, {"Time"=2.869999999999983, "delVelocity"=-0.7071067811865339}, {"Time"=2.8799999999999826, "delVelocity"=-0.7071067811865284}, {"Time"=2.8899999999999824, "delVelocity"=-0.7071067811865339}, {"Time"=2.899999999999982, "delVelocity"=-0.7071067811865339}, {"Time"=2.909999999999982, "delVelocity"=-0.7071067811865284}, {"Time"=2.9199999999999817, "delVelocity"=-0.7071067811865339}, {"Time"=2.9299999999999815, "delVelocity"=-0.7071067811865339}, {"Time"=2.9399999999999813, "delVelocity"=-0.7071067811865339}, {"Time"=2.949999999999981, "delVelocity"=-0.7071067811865284}, {"Time"=2.959999999999981, "delVelocity"=-0.7071067811865339}, {"Time"=2.9699999999999807, "delVelocity"=-0.7071067811865339}, {"Time"=2.9799999999999804, "delVelocity"=-0.7071067811865339}, {"Time"=2.9899999999999802, "delVelocity"=-0.7071067811865284}, {"Time"=2.99999999999998, "delVelocity"=-0.7071067811865339}, {"Time"=3.00999999999998, "delVelocity"=-0.7071067811865339}, {"Time"=3.0199999999999796, "delVelocity"=-0.7071067811865311}, {"Time"=3.0299999999999794, "delVelocity"=-0.7071067811865311}, {"Time"=3.039999999999979, "delVelocity"=-0.7071067811865339}, {"Time"=3.049999999999979, "delVelocity"=-0.7071067811865311}, {"Time"=3.0599999999999787, "delVelocity"=-0.7071067811865311}, {"Time"=3.0699999999999785, 
